vi "detectAndTransExtremePoint.vi"(5 "Col":u16, 7 "Row":u16, 8 "Level3 Memory":refnum<k21>, 9 "Level2 Memory":refnum<k21>, 10 "Level1 Memory":refnum<k21>, 11 "Width":u16) -> (2 "isExtreme?":bool)   [LabVIEW 2016]
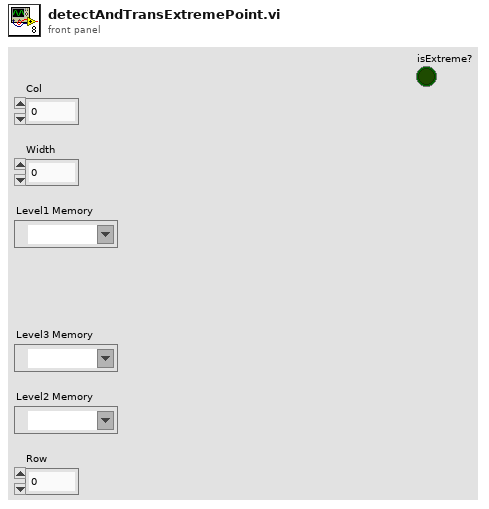
[diagram p1: front panel]
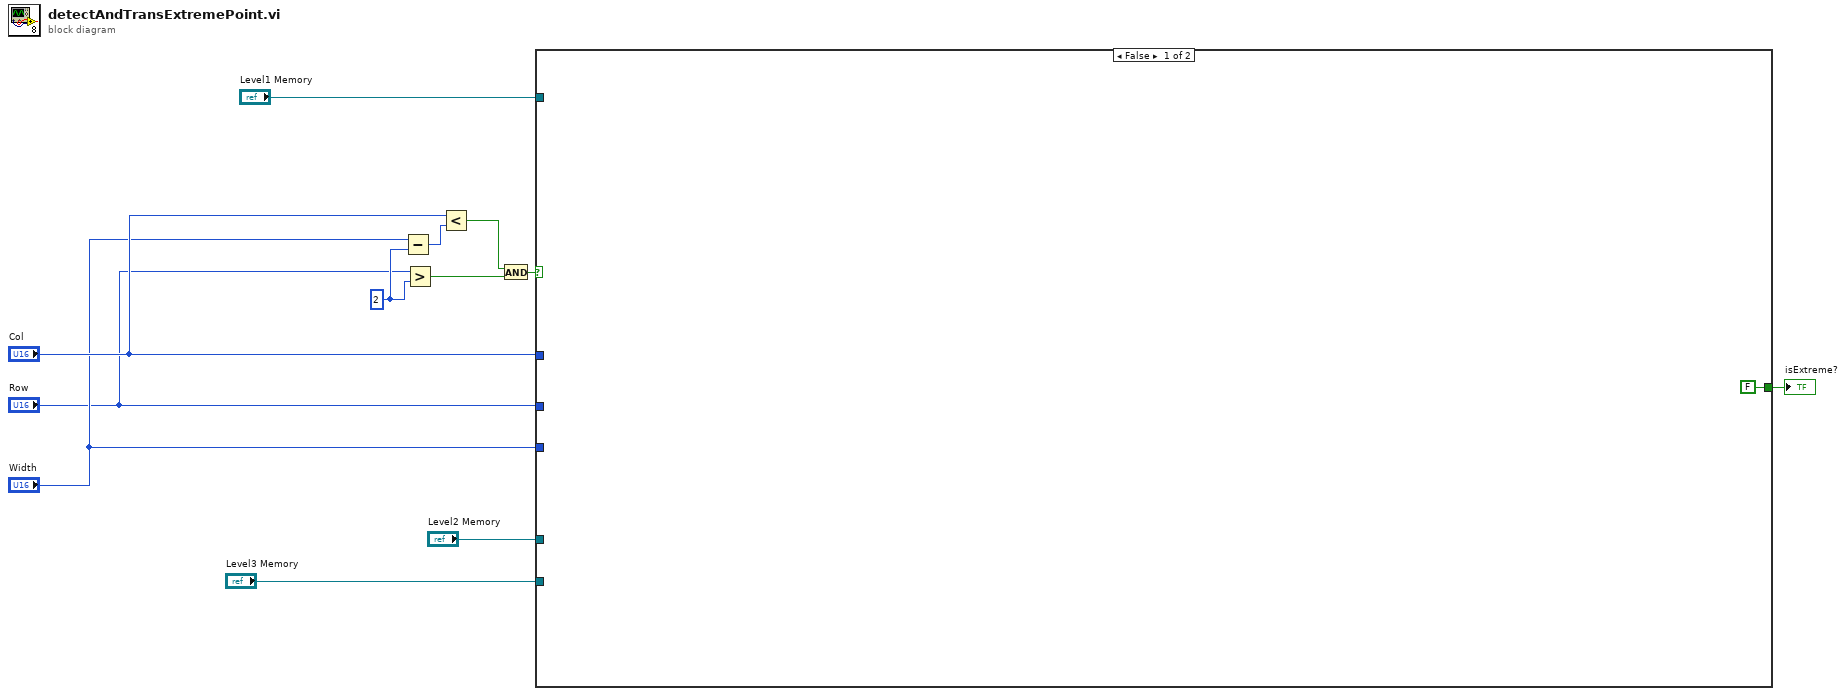
[diagram p0: block diagram]
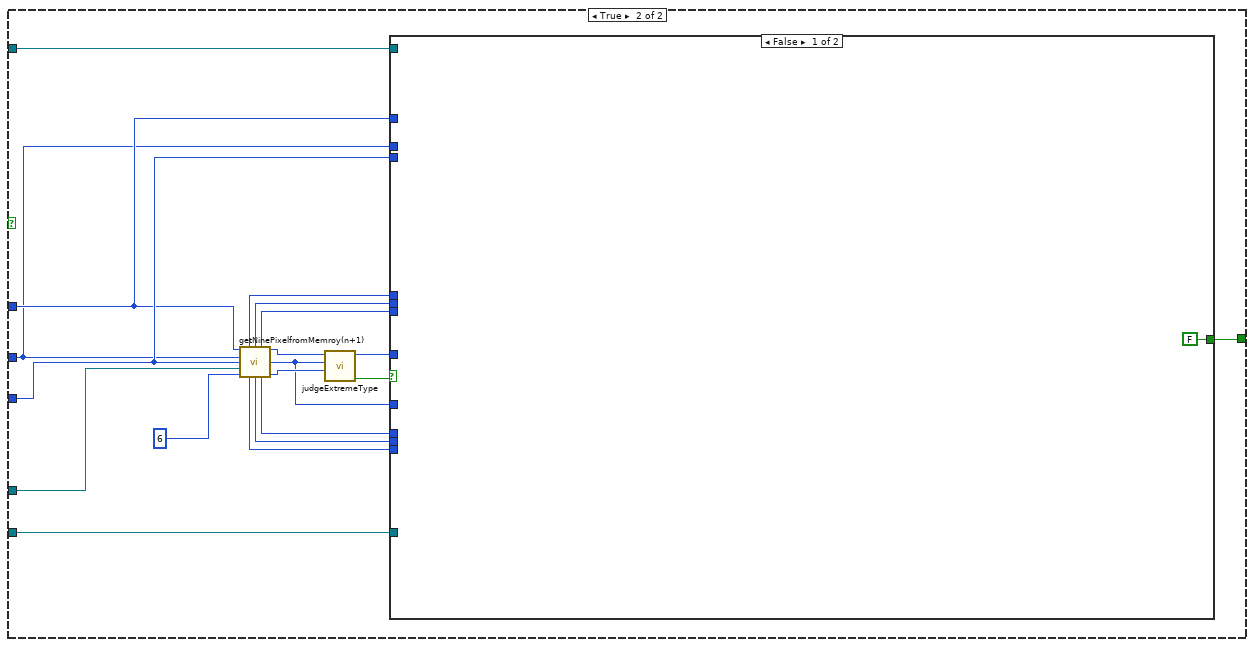
[diagram p2: hidden frame]
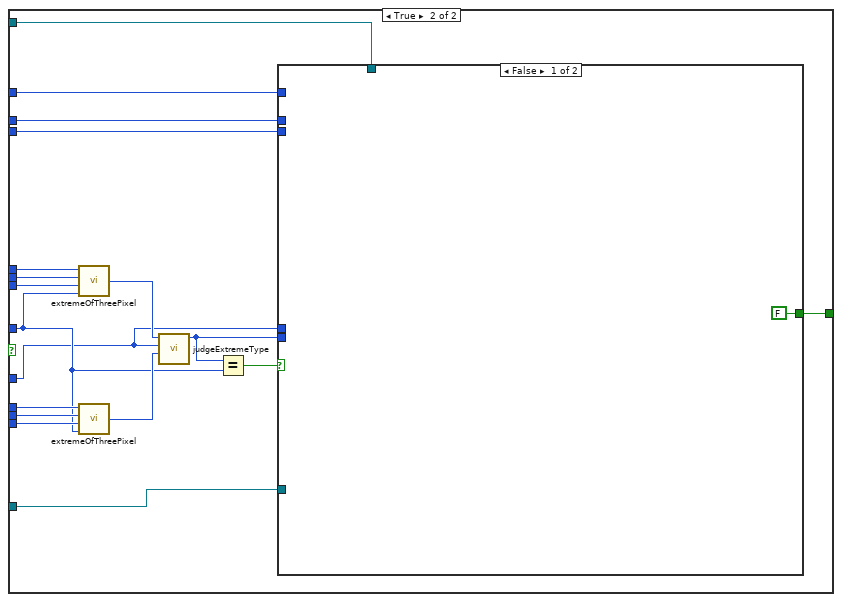
[diagram p3: hidden frame]
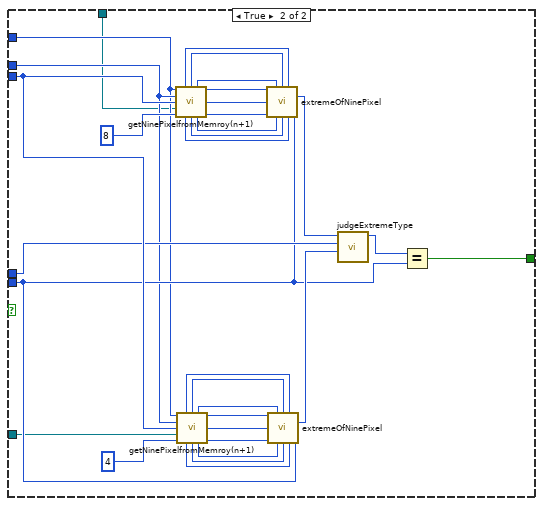
[diagram p4: hidden frame]
diagram:
  w4 = u16 2 ("y")
  n1 = Subtract(x="Width", y=w4) -> (x-y=w3:u16)
  n2 = Greater?(x="Row", y=w4) -> (0:w9:bool)
  n3 = Less?(x="Col", y=w3) -> (x < y?=w8:bool)
  n4 = And(x=w8, y=w9) -> (x .and. y?=w7:bool)
  n5 = case shown="False" w7 {
    tunnel: "Width" -> [_ w20]
    tunnel: "Row" -> [_ w18]
    tunnel: "Col" -> [_ w19]
    tunnel: "Level2 Memory" -> [_ w17]
    tunnel: "Level3 Memory" -> [_ w16]
    tunnel: "Level1 Memory" -> [_ w15]
    tunnel: [FALSE w14] -> w1
    frame False {
    }
    frame True {
      n6 = call "getNinePixelfromMemroy(n+1).vi"("col"=w19, "row"=w18, "Width"=w20, "Memory In"=w17, "divider"=u8 6) -> ("1"=w27:i8, "2"=w28:i8, "3"=w29:i8, "4"=w31:i8, "5"=w21:i8, "9"=w24:i8, "8"=w25:i8, "7"=w26:i8, "6"=w30:i8)  [unwired: 2 in]
      n7 = call "judgeExtremeType.vi"("next"=w30, "current"=w21, "previous"=w31) -> ("isExtreme?"=w22:bool, "extreme Type"=w23:u8)  [unwired: 7 in]
      n8 = case shown="False" w22 {
        tunnel: w29 -> [_ w51]
        tunnel: w28 -> [_ w50]
        tunnel: w27 -> [_ w49]
        tunnel: w26 -> [_ w48]
        tunnel: w25 -> [_ w47]
        tunnel: w24 -> [_ w46]
        tunnel: w23 -> [_ w43]
        tunnel: w21 -> [_ w37]
        tunnel: w20 -> [_ w41]
        tunnel: w18 -> [_ w40]
        tunnel: w19 -> [_ w39]
        tunnel: w16 -> [_ w36]
        tunnel: w15 -> [_ w35]
        tunnel: [FALSE w34] -> w14
        frame False {
        }
        frame True {
          n9 = call "extremeOfThreePixel.vi"("extreme Type"=w43, "3"=w51, "2"=w50, "1"=w49) -> ("extreme out"=w45:i8)
          n10 = call "extremeOfThreePixel.vi"("extreme Type"=w43, "3"=w46, "2"=w47, "1"=w48) -> ("extreme out"=w44:i8)
          n11 = call "judgeExtremeType.vi"("next"=w44, "current"=w37, "previous"=w45) -> ("extreme Type"=w38:u8)  [unwired: 7 in, 1 out]
          n12 = Equal?(x=w38, y=w43) -> (x = y?=w42:bool)
          n13 = case shown="False" w42 {
            tunnel: w41 -> [_ w63]
            tunnel: w40 -> [_ w57]
            tunnel: w39 -> [_ w56]
            tunnel: w38 -> [_ w58]
            tunnel: w37 -> [_ w61]
            tunnel: w36 -> [_ w55]
            tunnel: w35 -> [_ w54]
            tunnel: [FALSE w53] -> w34
            frame False {
            }
            frame True {
              n14 = call "getNinePixelfromMemroy(n+1).vi"("col"=w56, "row"=w57, "Width"=w63, "Memory In"=w54, "divider"=u8 8) -> ("1"=w80:i8, "2"=w81:i8, "3"=w82:i8, "4"=w79:i8, "5"=w78:i8, "9"=w74:i8, "8"=w75:i8, "7"=w76:i8, "6"=w77:i8)  [unwired: 2 in]
              n15 = call "getNinePixelfromMemroy(n+1).vi"("col"=w56, "row"=w57, "Width"=w63, "Memory In"=w55, "divider"=u8 4) -> ("1"=w70:i8, "2"=w71:i8, "3"=w72:i8, "4"=w69:i8, "5"=w68:i8, "9"=w64:i8, "8"=w65:i8, "7"=w66:i8, "6"=w67:i8)  [unwired: 2 in]
              n16 = call "extremeOfNinePixel.vi"("4"=w79, "3"=w82, "2"=w81, "1"=w80, "5"=w78, "6"=w77, "7"=w76, "8"=w75, "9"=w74, "extreme Type"=w58) -> ("extreme out"=w62:i8)  [unwired: 5 in]
              n17 = call "extremeOfNinePixel.vi"("4"=w69, "3"=w72, "2"=w71, "1"=w70, "5"=w68, "6"=w67, "7"=w66, "8"=w65, "9"=w64, "extreme Type"=w58) -> ("extreme out"=w60:i8)  [unwired: 5 in]
              n18 = call "judgeExtremeType.vi"("next"=w60, "current"=w61, "previous"=w62) -> ("extreme Type"=w59:u8)  [unwired: 7 in, 1 out]
              n19 = Equal?(x=w59, y=w58) -> (x = y?=w53:bool)
            }
          }
        }
      }
    }
  }
  "isExtreme?" <- w1
